vi "Get Answers Data Length.vi"(8 "error in (no error)":errorcluster, 11 "length":u32) -> (0 "error out":errorcluster, 2 "function return":bool, 3 "length out":u32)   [LabVIEW 2015, in "XGL_DPP.lvlib"]
doc: "EXTERN DECLSPEC bool CALL_CONV GetAnswersDataLength(unsigned int& length);"
uses:
  XGL_DPP.lvlib
  XGL_DPP.dll
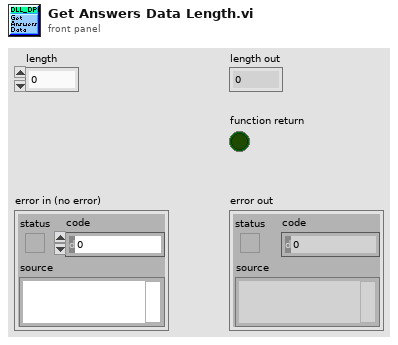
[diagram p1: front panel]
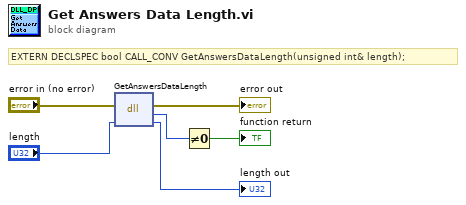
[diagram p0: block diagram]
diagram:
  # "EXTERN DECLSPEC bool CALL_CONV GetAnswersDataLength(unsigned int& length);"
  n1 = dll-call lib="D:/Users/XRF/Desktop/Dante_acquire4/libs/Dante/XGL_DPP.*" fn="GetAnswersDataLength"(error in="error in (no error)", "length"="length") -> (error out=→"error out":errorcluster, "return type"=w5:u8, "length"=→"length out":u32)  [unwired: 2 in, 1 out]
  n2 = Not Equal To 0?(x=w5) -> (x != 0?=→"function return":bool)
